vi "故障码字段定义.vi"(11 "故障代码":u16(ring)) -> (3 "字符串":string)   [LabVIEW 2016, in "斯坦道总氮.lvlib"]
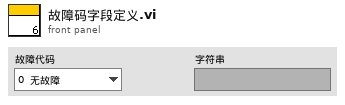
[diagram p1: front panel]
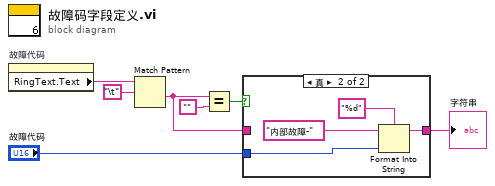
[diagram p0: block diagram]
diagram:
  n1 = property on="故障代码" class="Ring (严格)"() -> ("RingText.Text"=w4:string)  [unwired: 2 in, 2 out]
  n2 = Match Pattern(string=w4, regular expression="\t") -> (after substring=w2:string)  [unwired: 1 in, 3 out]
  n3 = Equal?(x=w2, y="") -> (x = y?=w6:bool)
  n4 = case shown="真" w6 {
    tunnel: [w8 w10] -> w5
    tunnel: w2 -> [w8 _]
    tunnel: "故障代码" -> [_ w9]
    frame False {
    }
    frame True {
      n5 = Format Into String(format string="%d" ("格式字符串"), initial string="内部故障-" ("工作状态"), w9) -> (resulting string=w10:string)  [unwired: 1 in, 1 out]
    }
  }
  "字符串" <- w5
